vi "Run Service.vi"() -> ()   [LabVIEW 2019, in "MicronGRPCGeneratedServer.lvlib"]
uses:
  MicronGRPCGeneratedServer.lvlib
  <vilib>/gRPC/LabVIEW gRPC Servicer/Servicer/Servicer.lvclass/Servicer.ctl
  <vilib>/gRPC/LabVIEW gRPC Servicer/ServiceBase/ServiceBase.lvclass
  <vilib>/gRPC/LabVIEW gRPC Servicer/Servicer/Servicer.lvclass
panel:
  in  "Async [T] / Sync [F]":bool
  out "Listening Port":i32
  in  "Stop":bool
  in  "Server Address":string="localhost:50051"
  in  "Server Certificate File (.crt)":path
  in  "Server Key File (.key)":path
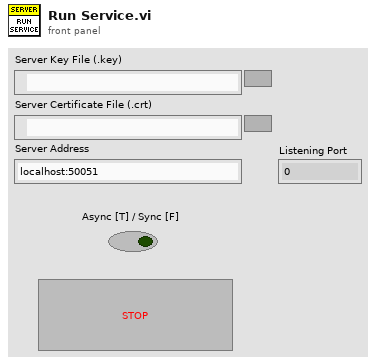
[diagram p1: front panel]
types:
  T1 = enum32{"Invalid", "Standard", "Closed", "Hidden", "Minimized", "Maximized"}
  T2 = typedef "grpc-lvsupport-release.lvlib/grpcId.ctl" = u64
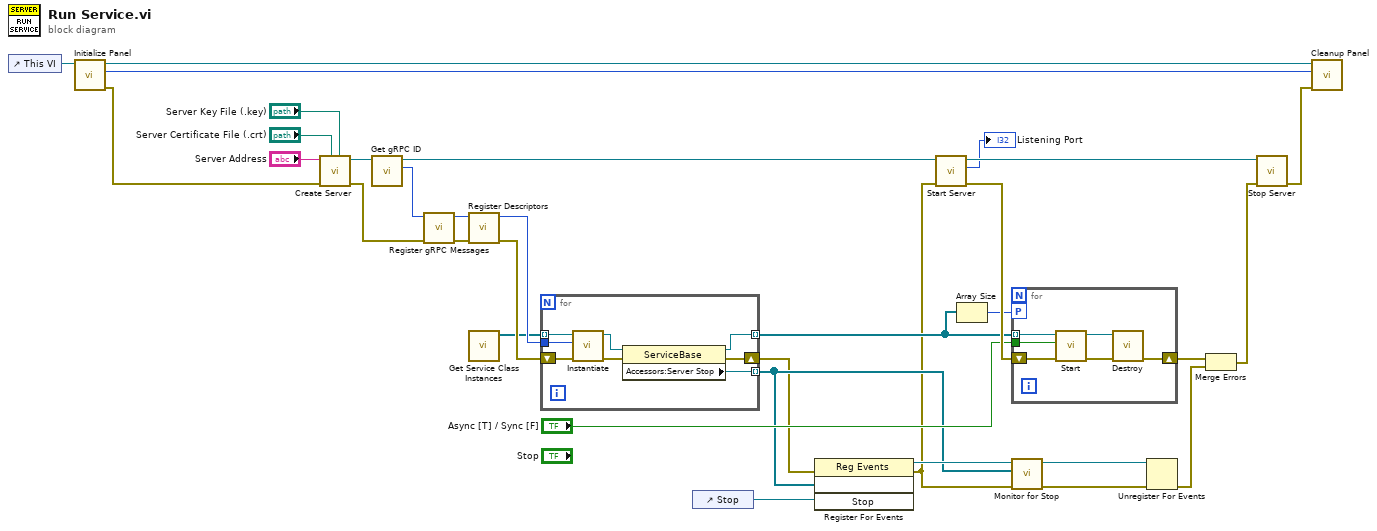
[diagram p0: block diagram]
diagram:
  n1 = control-ref of="This VI"() -> (w4:refnum<vi>)
  n2 = call "Initialize Panel.vi"("vi reference in"=w4) -> ("error out"=w5:errorcluster, "initial window state"=w2:T1, "vi reference out"=w3:refnum<vi>)  [unwired: 8 in]
  n3 = call <vilib>:"Create Server.vi"("Server Key File (.key)"="Server Key File (.key)", "Server Certificate File (.crt)"="Server Certificate File (.crt)", "error in"=w5, "Server Address"="Server Address") -> ("error out"=w25:errorcluster, "gRPC server out"=w27:refnum<class "Servicer.lvclass">)  [unwired: 6 in]
  n4 = call <vilib>:"Get gRPC ID.vi"("gRPC server in"=w27) -> ("gRPC ID"=w26:T2, "gRPC server out"=w22:refnum<class "Servicer.lvclass">)  [unwired: 9 in]
  n5 = call "Register gRPC Messages.vi"("error in (no error)"=w25, "gRPC ID"=w26) -> ("error out"=w24:errorcluster, "gRPC ID Out"=w23:T2)  [unwired: 8 in]
  n6 = call "Register Descriptors.vi"("error in (no error)"=w24, "gRPC ID"=w23) -> ("error out"=w21:errorcluster, "gRPC ID Out"=w20:T2)  [unwired: 8 in]
  n7 = call "Get Service Class Instances.vi"() -> ("service instances"=w19:refnum<class "ServiceBase.lvclass">[])  [unwired: 11 in]
  n8 = for {
    tunnel: [w37] -> w14 mode=indexing
    tunnel: w20 -> [w35]
    shift-right: [w34] -> w13
    shift-left: w21 -> [w36]
    tunnel: w19 -> [w40] mode=indexing
    tunnel: [w39] -> w15 mode=indexing
    n9 = call-dynamic "Instantiate.vi"("error in"=w36, "gRPCid"=w35, "gRPC service in"=w40) -> ("error out"=w38:errorcluster, "gRPC service out"=w41:refnum<class "ServiceBase.lvclass">)  [unwired: 7 in]
    n10 = property class="ServiceBase"(reference=w41, error in=w38) -> (reference out=w39:refnum<class "ServiceBase.lvclass">, error out=w34:errorcluster, "Accessors:Server Stop"=w37:refnum<user-event>)
  }
  n11 = control-ref of="Stop"() -> (w9:refnum<vi>)
  n12 = register-events(error in=w13, w14, w9) -> (reference out=w29:refnum<event-registration>, error out=w12:errorcluster)  [unwired: 1 in]
  n13 = call <vilib>:"Start Server.vi"("error in"=w12, "gRPC server in"=w22) -> ("error out"=w18:errorcluster, "Listening Port"=→"Listening Port":i32, "gRPC server out"=w33:refnum<class "Servicer.lvclass">)  [unwired: 7 in]
  n14 = Array Size(array=w15) -> (size(s)=w16:i32)
  n15 = for {
    tunnel: w15 -> [w45] mode=indexing
    tunnel: "Async [T] / Sync [F]" -> [w43]
    workers-P: w16 -> [_]
    shift-right: [w42] -> w11
    shift-left: w18 -> [w44]
    n16 = call-dynamic "Start.vi"("error in"=w44, "ASync [T]"=w43, "gRPC service in"=w45) -> ("error out"=w46:errorcluster, "gRPC service out"=w47:refnum<class "ServiceBase.lvclass">)  [unwired: 7 in]
    n17 = call-dynamic "Destroy.vi"("error in"=w46, "gRPC service in"=w47) -> ("error out"=w42:errorcluster)  [unwired: 8 in, 1 out]
  }
  n18 = call "Monitor for Stop.vi"("error in (no error)"=w12, "service stop events"=w14, "Event Registration Refnum in"=w29) -> ("error out"=w6:errorcluster, "Event Registration Refnum out"=w8:refnum<event-registration>)  [unwired: 7 in]
  n19 = Unregister For Events(event registration refnum=w8, error in=w6) -> (error out=w7:errorcluster)
  n20 = Merge Errors(w11, w7) -> (w10:errorcluster)
  n21 = call <vilib>:"Stop Server.vi"("error in"=w10, "gRPC server in"=w33) -> ("error out"=w1:errorcluster)  [unwired: 9 in]
  n22 = call "Cleanup Panel.vi"("error in (no error)"=w1, "initial window state"=w2, "vi reference in"=w3) -> ()  [unwired: 7 in, 2 out]
